vi "Add Transaction.vi"(8 "Error In (no error)":errorcluster, 10 "Transaction":T1, 11 "DB Operator In":refnum<class "DB Operator.lvclass">) -> (0 "Error Out":errorcluster, 3 "DB Operator Out":refnum<class "DB Operator.lvclass">)   [LabVIEW 2023, in "DB Operator.lvclass"]
uses:
  DB Operator.lvclass
  Public/Ctrls/DB Controls/Transaction.ctl
  DB Operator.lvclass/DB Operator.ctl
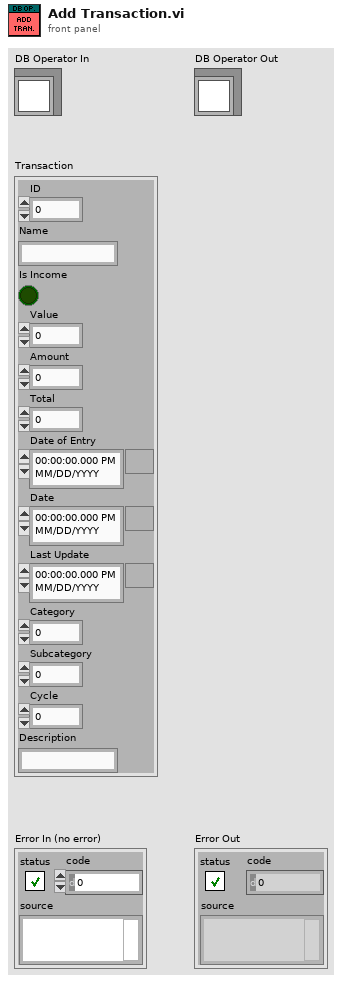
[diagram p1: front panel]
types:
  T1 = typedef "DB Operator.lvclass/Transaction.ctl" = cluster{"ID":u64, "Name":string, "Is Income":bool, "Value":dbl, "Amount":dbl, "Total":dbl, "Date of Entry":timestamp, "Date":timestamp, "Last Update":timestamp, "Category":u32, "Subcategory":u32, "Cycle":u32, "Description":string}
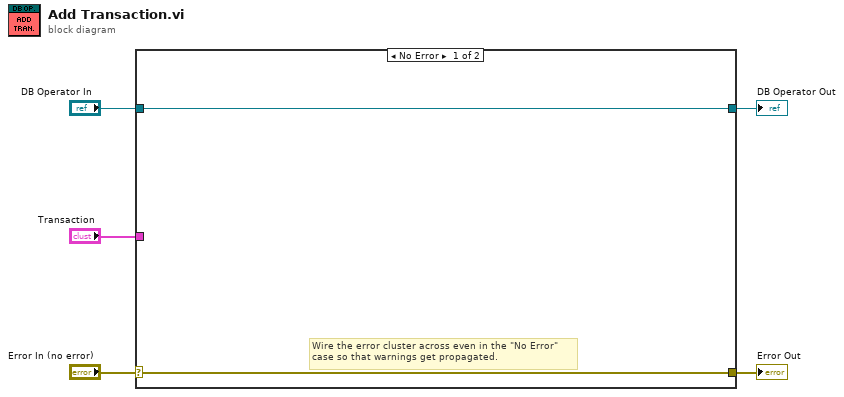
[diagram p0: block diagram]
diagram:
  n1 = case shown="No Error" "Error In (no error)" {
    selector: "Error In (no error)" -> [w6 w9]
    tunnel: [w6 w9] -> w4
    tunnel: [w7 w8] -> w2
    tunnel: "DB Operator In" -> [w7 w8]
    tunnel: "Transaction" -> [_ _]
    frame No Error {
      # "Wire the error cluster across even in the \"No Error\"\ncase so that warnings get propagated."
    }
    frame Error {
    }
  }
  "Error Out" <- w4
  "DB Operator Out" <- w2
